vi "AttenCorr.vi"(4 "sound speed":dbl=1.5 format="%.2f", 5 "Offset":i32=32, 6 "Step size":i32=8, 7 "Attenuation (db/ cm MHz)":dbl=0.5 format="%.2f", 8 "Sampling Freq (MHz)":i32=50, 9 "Center Freq":dbl=5.75 format="%.2f", 10 "ROIs in x":i32) -> (0 "slope correction":dbl[](array[numeric]) format="%.2f", 2 "midband correction":dbl[](array[numeric]) format="%.2f")   [LabVIEW 2022 SP3]
panel:
  # "used to generate attenuation correction. Defaults are for TPI images. Set step size to 1 and offset to zero for normal RF data. Offsset means the location of center of first TPI window in terms of RF pts, normally 32. Step size is increment of sliding window."
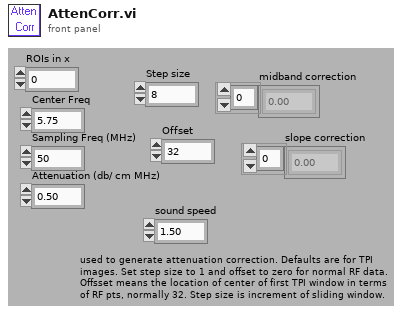
[diagram p1: front panel]
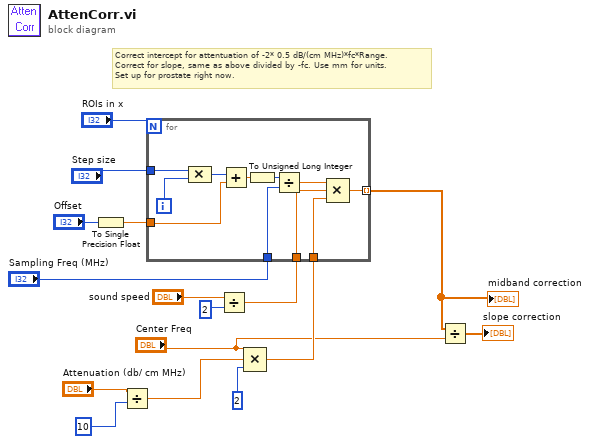
[diagram p0: block diagram]
diagram:
  # "Correct intercept for attentuation of -2* 0.5 dB/(cm MHz)*fc*Range.\nCorrect for slope, same as above divided by -fc. Use mm for units. \nSet up for prostate right now."
  n1 = To Single Precision Float(number="Offset") -> (single precision float=w5:sgl)
  n2 = Divide(x="Attenuation (db/ cm MHz)", y=10) -> (x/y=w9:dbl)
  n3 = Divide(x="sound speed", y=2) -> (x/y=w2:dbl)
  n4 = Compound Arithmetic op=MULTIPLY("Center Freq", w9, 2) -> (w15:dbl)
  n5 = for {
    N: "ROIs in x" -> [_]
    tunnel: "Sampling Freq (MHz)" -> [w24]
    tunnel: w2 -> [w22]
    tunnel: [w20] -> w14 mode=indexing
    tunnel: w15 -> [w21]
    tunnel: w5 -> [w19]
    tunnel: "Step size" -> [w18]
    i -> [w27]
    n6 = Compound Arithmetic op=MULTIPLY(w18, w27) -> (w26:i32)
    n7 = Add(x=w26, y=w19) -> (x+y=w25:sgl)
    n8 = To Unsigned Long Integer(number=w25) -> (unsigned 32bit integer=w17:u32)
    n9 = Divide(x=w17, y=w24) -> (x/y=w23:dbl)
    n10 = Compound Arithmetic op=MULTIPLY(w23, w22, w21) -> (w20:dbl)
  }
  "midband correction" <- w14
  n11 = Divide(x=w14, y="Center Freq") -> (x/y=→"slope correction":dbl[])
